vi "Set Processes Lookup.vi"(10 "Processes Lookup":T1[](array[typedef]), 11 "Process in":refnum<class "Process.lvclass">) -> (3 "Process out":refnum<class "Process.lvclass">)   [LabVIEW 2019, in "TimingDRV Engine.lvlib" / "Process.lvclass"]
uses:
  Process.lvclass
  TypeDefs/Process Lookup.ctl
  TypeDefs/Message.ctl
  TypeDefs/Update.ctl
  Process.lvclass/Process.ctl
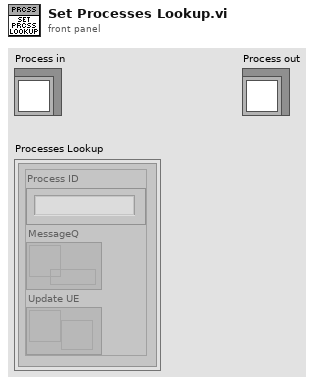
[diagram p1: front panel]
types:
  T1 = typedef "TimingDRV Engine.lvlib/Process.lvclass/Process Lookup.ctl" = cluster{"Process ID":string, "MessageQ":refnum<queue>, "Update UE":refnum<user-event>}
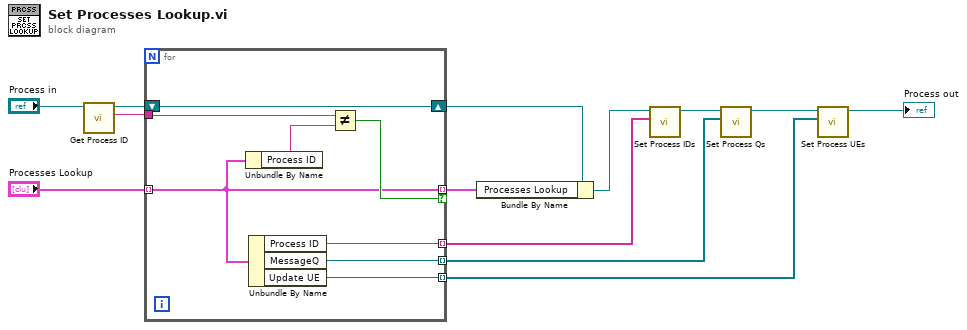
[diagram p0: block diagram]
diagram:
  n1 = call "Get Process ID.vi"("CD_Process in"="Process in") -> ("Process ID"=w11:string, "CD_Process out"=w10:refnum<class "Process.lvclass">)  [unwired: 9 in]
  n2 = for {
    tunnel: "Processes Lookup" -> [w17] mode=indexing
    tunnel: w11 -> [w20]
    tunnel: [w17] -> w8 mode=indexing if=w19
    shift-right: [w18] -> w9
    shift-left: w10 -> [w18]
    tunnel: [w16] -> w6 mode=indexing
    tunnel: [w15] -> w4 mode=indexing
    tunnel: [w14] -> w3 mode=indexing
    n3 = Unbundle By Name(w17) -> ("Process ID"=w21:string)
    n4 = Unbundle By Name(w17) -> ("Process ID"=w16:string, "MessageQ"=w15:refnum<queue>, "Update UE"=w14:refnum<user-event>)
    n5 = Not Equal?(x=w20, y=w21) -> (x != y?=w19:bool)
  }
  n6 = Bundle By Name(cluster=w9, "Processes Lookup"=w8) -> (w7:refnum<class "Process.lvclass">)
  n7 = call "Set Process IDs.vi"("Process IDs"=w6, "Process in"=w7) -> ("Process out"=w5:refnum<class "Process.lvclass">)  [unwired: 9 in]
  n8 = call "Set Process Qs.vi"("Process Qs"=w4, "Process in"=w5) -> ("Process out"=w2:refnum<class "Process.lvclass">)  [unwired: 9 in]
  n9 = call "Set Process UEs.vi"("Process UEs"=w3, "Process in"=w2) -> ("Process out"=→"Process out":refnum<class "Process.lvclass">)  [unwired: 9 in]
